vi "CheckUnique_检查唯一性.vi"(11 "SourceString":string[](array[string])) -> (2 "HasDuplication":bool, 3 "UniqueString":string[](array[string]))   [LabVIEW 2018]
panel:
  out "DuplicationString":string[](array[string])
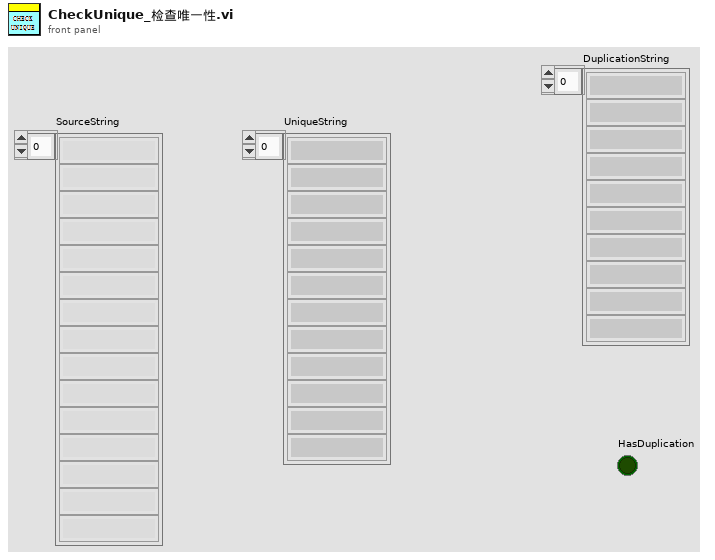
[diagram p1: front panel]
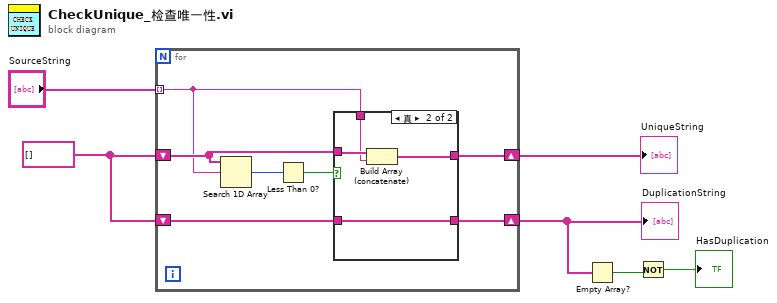
[diagram p0: block diagram]
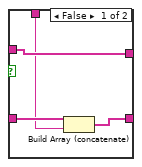
[diagram p2: hidden frame]
diagram:
  w4 = string[] [] ("SourceString")
  n1 = for {
    tunnel: "SourceString" -> [w10] mode=indexing
    shift-right: [w9] -> w5
    shift-left: w4 -> [w11]
    shift-right: [w7] -> w3
    shift-left: w4 -> [w8]
    n2 = Search 1D Array(1D array=w11, element=w10) -> (index of element=w13:i32)  [unwired: 1 in]
    n3 = Less Than 0?(x=w13) -> (x < 0?=w12:bool)
    n4 = case shown="真" w12 {
      tunnel: w11 -> [w17 w21]
      tunnel: [w17 w20] -> w9
      tunnel: w10 -> [w15 w19]
      tunnel: w8 -> [w16 w18]
      tunnel: [w14 w18] -> w7
      frame False {
        n5 = Build Array (concatenate)(w16, w15) -> (w14:string[])
      }
      frame True {
        n6 = Build Array (concatenate)(w21, w19) -> (w20:string[])
      }
    }
  }
  "UniqueString" <- w5
  "DuplicationString" <- w3
  n7 = Empty Array?(array=w3) -> (empty?=w2:bool)
  n8 = Not(x=w2) -> (.not. x?=→"HasDuplication":bool)
